vi "DetectActive Channels.vi"(8 "error in (no error)":errorcluster, 11 "resourcename in":string) -> (0 "error out":errorcluster, 2 "Array":u16[](array[numeric]), 3 "resourcename out":string)   [LabVIEW 2020, in "Tektronix MDO MSO DPO.lvclass"]
uses:
  Tektronix MDO MSO DPO.lvclass
  Tektronix DPO MSO 2000 4000 Series/Tektronix DPO MSO 2000 4000 Series.lvlib
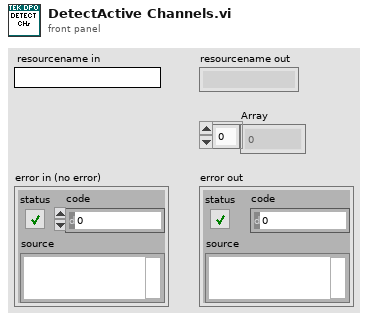
[diagram p1: front panel]
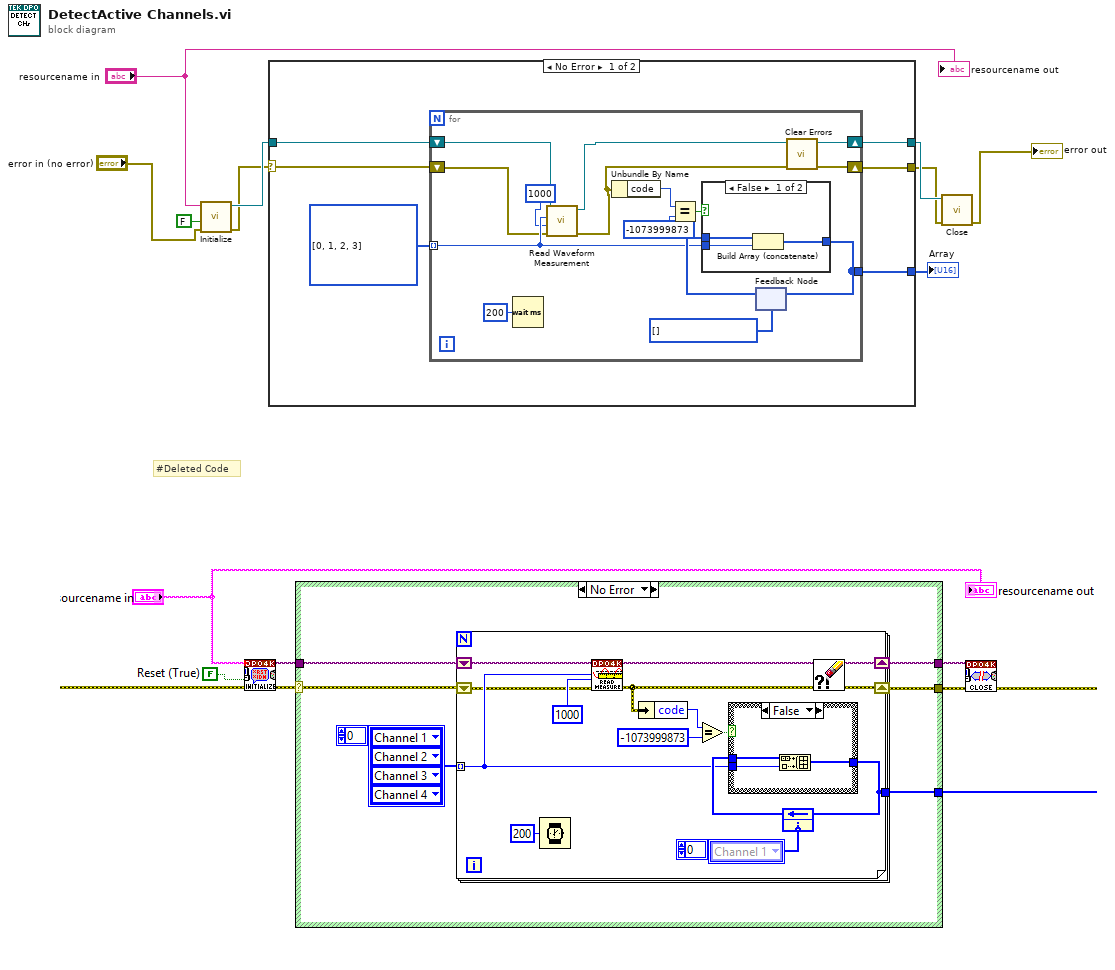
[diagram p0: block diagram]
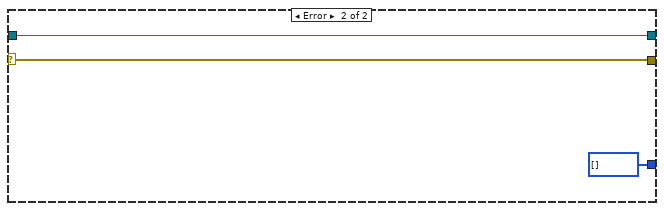
[diagram p3: hidden frame]
diagram:
  # "#Deleted Code"
  n1 = call "Initialize.vi"("error in (no error)"="error in (no error)", "Reset (True)"=FALSE, "VISA resource name"="resourcename in") -> ("error out"=w4:errorcluster, "VISA resource name out"=w6:refnum<visa-resource-name>)  [unwired: 7 in]
  n2 = case shown="No Error" w4 {
    selector: w4 -> [w10 w36]
    tunnel: w6 -> [w15 w35]
    tunnel: [w14 w35] -> w3
    tunnel: [w13 w36] -> w2
    tunnel: [w11 u16[] []] -> w9
    frame No Error {
      w12 = u16[] [0, 1, 2, 3] items=["Channel 1", "Channel 2", "Channel 3", "Channel 4", "Math", "Reference 1", "Reference 2", "Reference 3", "Reference 4", "D0", "D1", "D2", "D3", "D4", "D5", "D6", "D7", "D8", "D9", "D10", "D11", "D12", "D13", "D14", "D15", "Amplitude", "Frequency", "Phase", "Normal", "Average", "Maximum Peak Hold", "Minimum Peak Hold"]
      n3 = for {
        tunnel: w12 -> [w21] mode=indexing
        shift-right: [w18] -> w14
        shift-left: w15 -> [w19]
        shift-right: [w28] -> w13
        shift-left: w10 -> [w17]
        tunnel: [w22] -> w11
        w23 = u16[] [] items=["Channel 1", "Channel 2", "Channel 3", "Channel 4", "Math", "Reference 1", "Reference 2", "Reference 3", "Reference 4", "D0", "D1", "D2", "D3", "D4", "D5", "D6", "D7", "D8", "D9", "D10", "D11", "D12", "D13", "D14", "D15", "Amplitude", "Frequency", "Phase", "Normal", "Average", "Maximum Peak Hold", "Minimum Peak Hold"]
        n4 = Wait (ms)(milliseconds to wait=u32 200) -> ()  [unwired: 1 out]
        n5 = call "Read Waveform Measurement.vi"("error in (no error)"=w17, "Maximum Time (10000ms)"=u32 1000, "Channel (0: Channel 1)"=w21, "VISA resource name"=w19) -> ("error out"=w16:errorcluster, "VISA resource name out"=w18:refnum<visa-resource-name>)  [unwired: 5 in, 1 out]
        n6 = Unbundle By Name(w16) -> ("code"=w27:i32)
        n7 = Equal?(x=w27, y=-1073999873) -> (x = y?=w25:bool)
        n8 = feedback #1(w23) -> (w24:u16[])
        n9 = case shown="False" w25 {
          tunnel: w21 -> [w31 _]
          tunnel: w24 -> [w32 w33]
          tunnel: [w30 w33] -> w22
          frame False {
            n10 = Build Array (concatenate)(w32, w31) -> (w30:u16[])
          }
          frame True {
          }
        }
        n11 = feedback-in #1(w22) -> ()
        n12 = call <vilib>:"Clear Errors.vi"("error in (no error)"=w16) -> ("error out"=w28:errorcluster)  [unwired: 5 in, 1 out]
      }
    }
    frame Error {
    }
  }
  "Array" <- w9
  n13 = call "Close.vi"("error in (no error)"=w2, "VISA resource name"=w3) -> ("error out"=→"error out":errorcluster)  [unwired: 9 in]
  "resourcename out" <- "resourcename in"
